vi "Deney 3.2.vi"() -> ()   [LabVIEW 2018]
panel:
  out "Q0":bool
  out "2":bool
  out "1":bool
  out "3":bool
  out "4":bool
  out "5":bool
  out "6":bool
  out "Q2":bool
  out "Q1":bool
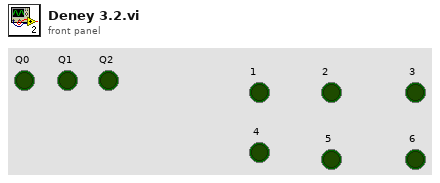
[diagram p1: front panel]
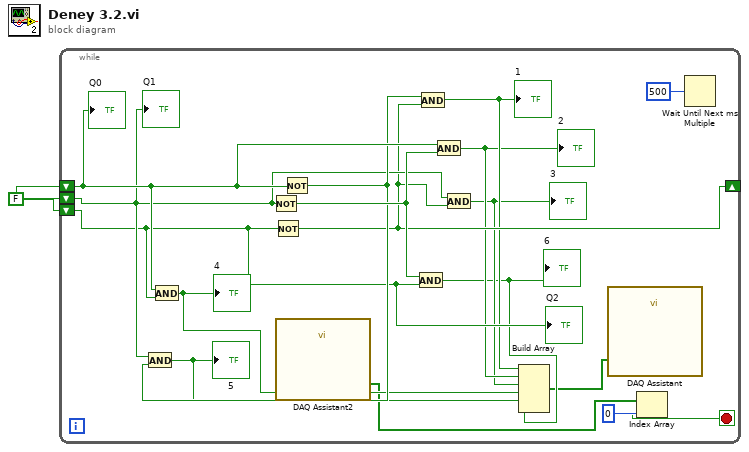
[diagram p0: block diagram]
diagram:
  w1 = FALSE
  n1 = while {
    shift-right: [w13] -> _
    shift-left: w1 -> [w17]
    shift-left: w1 -> [w14]
    shift-left: w1 -> [w12]
    stop <- w10 stop-if-true
    n2 = And(x=w17, y=w12) -> (x .and. y?=w6:bool)
    "4" <- w6
    n3 = Not(x=w14) -> (.not. x?=w16:bool)
    n4 = Not(x=w12) -> (.not. x?=w13:bool)
    n5 = call "DAQ Assistant2"() -> ("data"=w2:bool[])  [unwired: 17 in, 2 out]
    n6 = Not(x=w17) -> (.not. x?=w15:bool)
    n7 = And(x=w14, y=w15) -> (x .and. y?=w5:bool)
    "5" <- w5
    n8 = And(x=w16, y=w12) -> (x .and. y?=w4:bool)
    "6" <- w4
    n9 = And(x=w15, y=w13) -> (x .and. y?=w9:bool)
    "1" <- w9
    n10 = And(x=w17, y=w16) -> (x .and. y?=w8:bool)
    "2" <- w8
    n11 = And(x=w14, y=w13) -> (x .and. y?=w7:bool)
    "3" <- w7
    n12 = Build Array(w9, w8, w7, w6, w5, w4) -> (w3:bool[])
    n13 = call "DAQ Assistant"("data"=w3) -> ()  [unwired: 17 in, 2 out]
    n14 = Index Array(array=w2, index=0) -> (element=w10:bool)
    n15 = Wait Until Next ms Multiple(millisecond multiple=500) -> ()  [unwired: 1 out]
    "Q0" <- w17
    "Q2" <- w12
    "Q1" <- w14
  }
